vi "Construct Rx UDP.vi"(0 "custom device ref in":T6=18446744073709551615 format="%.0x", 1 "async loop rate hz":dbl, 5 "InstrumentHandle_board":u32, 7 "InstrumentHandle_port":u32, 9 "VL Configurations":T5(array[cluster]) {"VL Config"."FilterMode" items=["FDX_RX_VL_FLT_DIS", "FDX_RX_VL_FLT_ENA ", "FDX_RX_VL_FLT_ENA_INV"]; "VL Config"."VLBufSize" format="%.0x"; "VL Config"."VerificationMode" items=["FDX_RX_VL_CHECK_ENA_DEFAULT"=65535, "FDX_RX_VL_CHECK_REDMAM"=16, "DX_RX_VL_CHECK_TRAFIC"=8, "FDX_RX_VL_CHECK_FRAMESIZE"=4, "FDX_RX_VL_CHECK_SNINTEG"=2, "FDX_RX_VL_CHECK_INVPAC"=1, "FDX_RX_VL_CHECK_DISA"=0]}, 11 "error in (no error)":errorcluster, 12 "CommPort Payload":T1[](array[typedef]) {"Parameters"."encoding" items=["BNR", "BCD", "Discrete", "Signed_32", "Signed_64", "Float_32", "Float_64", "Opaque"]}) -> (4 "custom device ref out":T6=18446744073709551615 format="%.0x", 6 "Execution Unit Out":refnum<class "Rx UDP Execution Unit.lvclass">, 15 "error out":errorcluster)   [LabVIEW 2020, in "AIM ARINC 664 Engine.lvlib" / "Implementation.lvlib" / "Rx UDP Execution Unit.lvclass"]
uses:
  Rx UDP Execution Unit.lvclass
  Execution Unit/Execution Unit.lvclass
  Execution Unit Factory/Execution Unit Factory.lvclass
  <vilib>/NI VeriStand/Custom Device API/Custom Device Item Ref.ctl
  <vilib>/NI VeriStand/Custom Device API/Custom Device API.lvlib
  Program Files/National Instruments/LabVIEW 2024/instr.lib/AIM GmbH/_AIM 664/_controls/comm_verification_rx.ctl
  Program Files/National Instruments/LabVIEW 2024/instr.lib/AIM GmbH/_AIM 664/AIM664LV.lvlib
  Program Files/National Instruments/LabVIEW 2024/instr.lib/AIM GmbH/_AIM 664/_controls/comm_udp_rx.ctl
  Shared/Encoding (Arinc664).ctl
  Shared/rx_udp_payload_config.ctl
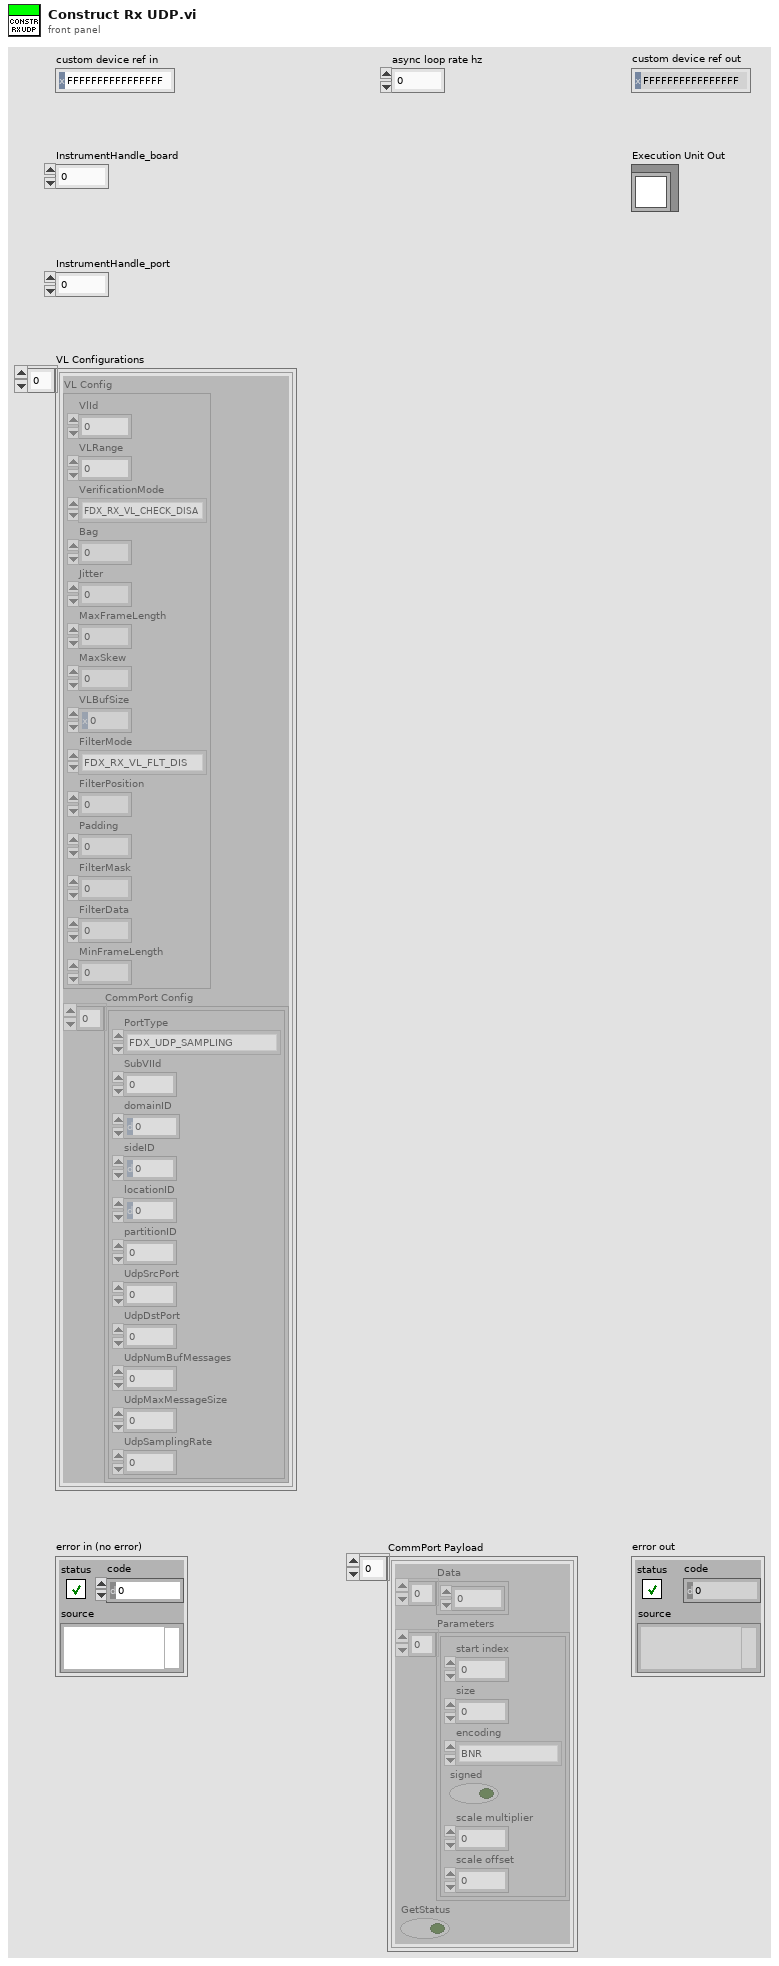
[diagram p1: front panel]
types:
  T1 = typedef "rx_udp_payload_config.ctl" = cluster{"Data":u8[], "Parameters":cluster{"start index":i32, "size":i32, "encoding":T2, "signed":bool, "scale multiplier":dbl, "scale offset":dbl}[], "GetStatus":bool}
  T2 = typedef "Encoding (Arinc664).ctl" = u16
  T3 = typedef "AIM664LV.lvlib/comm_verification_rx.ctl" = cluster{"VlId":u16, "VLRange":u32, "VerificationMode":u32, "Bag":u32, "Jitter":u32, "MaxFrameLength":u32, "MaxSkew":u32, "VLBufSize":u32, "FilterMode":u32, "FilterPosition":u32, "Padding":u32, "FilterMask":u32, "FilterData":u32, "MinFrameLength":u32}
  T4 = typedef "AIM664LV.lvlib/comm_udp_rx.ctl" = cluster{"PortType":enum16{"FDX_UDP_SAMPLING", "FDX_UDP_QUEUING"}, "SubVIId":u32, "domainID":u8, "sideID":u8, "locationID":u8, "partitionID":u8, "UdpSrcPort":u16, "UdpDstPort":u16, "UdpNumBufMessages":u32, "UdpMaxMessageSize":u32, "UdpSamplingRate":u32}
  T5 = cluster{"VL Config":T3, "CommPort Config":T4[]}[]
  T6 = typedef "Custom Device API.lvlib/Custom Device Item Ref.ctl" = u64
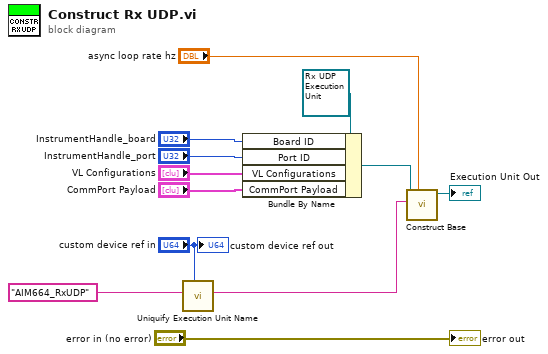
[diagram p0: block diagram]
diagram:
  n1 = call "Uniquify Execution Unit Name.vi"("custom device ref"="custom device ref in", "execution unit name"="AIM664_RxUDP") -> ("execution unit name out"=w10:string)  [unwired: 9 in]
  n2 = Bundle By Name(cluster=refnum<class "Rx UDP Execution Unit.lvclass"> refnum ("Communication Bus Template Interfaces:Implementation.lvlib:Rx UDP Execution Unit.lvclass"), "Board ID"="InstrumentHandle_board", "Port ID"="InstrumentHandle_port", "VL Configurations"="VL Configurations", "CommPort Payload"="CommPort Payload") -> (w12:refnum<class "Rx UDP Execution Unit.lvclass">)
  n3 = call "Construct Base.vi"("Execution Unit Implementation (default object)"=w12, "identifier"=w10, "async loop rate hz"="async loop rate hz") -> ("Execution Unit Out"=→"Execution Unit Out":refnum<class "Rx UDP Execution Unit.lvclass">)  [unwired: 6 in, 1 out]
  "error out" <- "error in (no error)"
  "custom device ref out" <- "custom device ref in"
